vi "多参数据转列表.vi"(7 "参数名":string, 11 "测量数据块":T1) -> (3 "添加的数组":string[][](array[string]))   [LabVIEW 2016, in "斯坦道仪器.lvlib"]
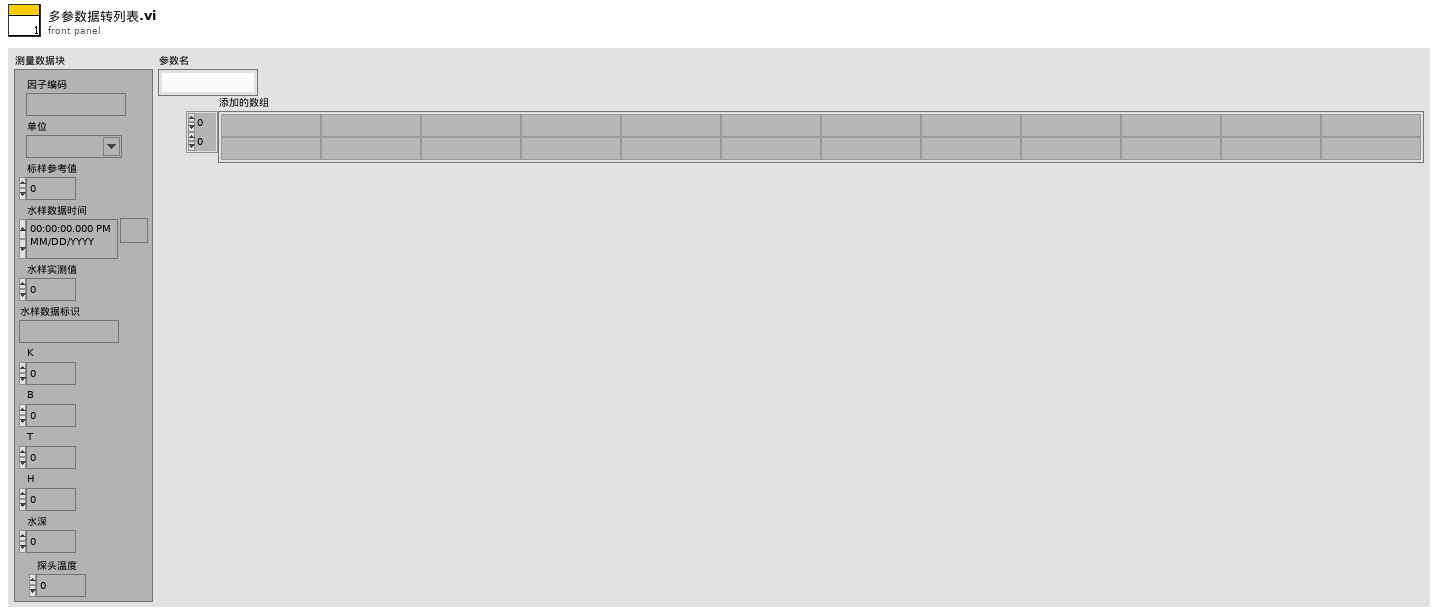
[diagram p1: front panel]
types:
  T1 = cluster{"因子编码":string, "单位":string, "标样参考值":sgl, "水样数据时间":timestamp, "水样实测值":sgl, "水样数据标识":string, "K":sgl, "B":sgl, "T":sgl, "H":sgl, "水深":sgl, "探头温度":sgl}
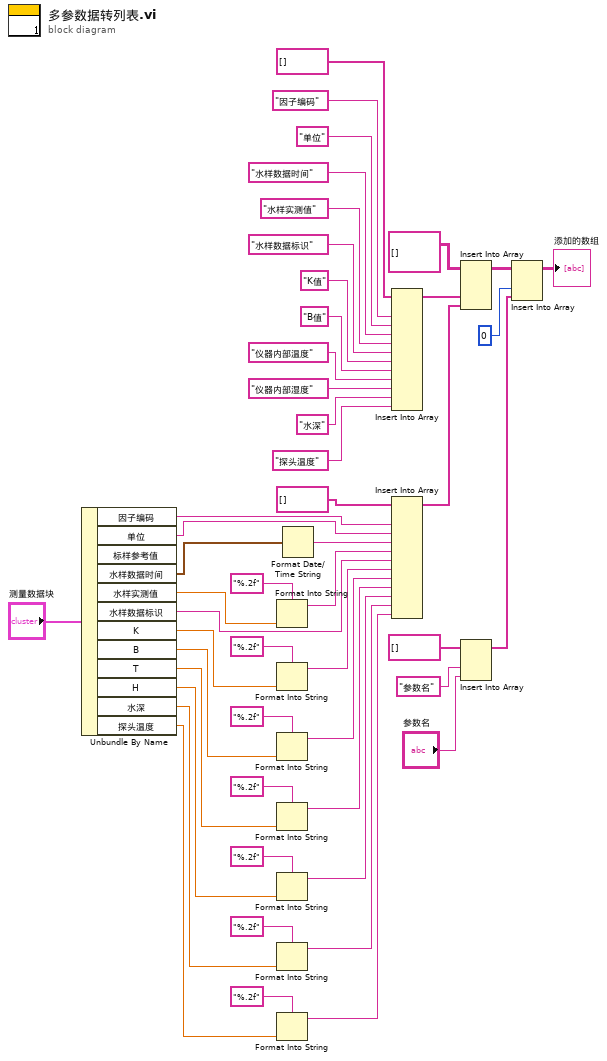
[diagram p0: block diagram]
diagram:
  n1 = Unbundle By Name("测量数据块") -> ("因子编码"=w31:string, "单位"=w30:string, "水样数据时间"=w29:timestamp, "水样实测值"=w28:sgl, "水样数据标识"=w27:string, "K"=w21:sgl, "B"=w20:sgl, "T"=w19:sgl, "H"=w18:sgl, "水深"=w17:sgl, "探头温度"=w2:sgl)  [unwired: 1 out]
  n2 = Format Into String(format string="%.2f" ("格式字符串"), w28) -> (resulting string=w47:string)  [unwired: 2 in, 1 out]
  n3 = Format Into String(format string="%.2f" ("格式字符串"), w21) -> (resulting string=w16:string)  [unwired: 2 in, 1 out]
  n4 = Format Into String(format string="%.2f" ("格式字符串"), w20) -> (resulting string=w15:string)  [unwired: 2 in, 1 out]
  n5 = Format Into String(format string="%.2f" ("格式字符串"), w19) -> (resulting string=w14:string)  [unwired: 2 in, 1 out]
  n6 = Format Into String(format string="%.2f" ("格式字符串"), w18) -> (resulting string=w13:string)  [unwired: 2 in, 1 out]
  n7 = Format Into String(format string="%.2f" ("格式字符串"), w17) -> (resulting string=w12:string)  [unwired: 2 in, 1 out]
  n8 = Format Into String(format string="%.2f" ("格式字符串"), w2) -> (resulting string=w1:string)  [unwired: 2 in, 1 out]
  n9 = Format Date/Time String(seconds (now)=w29) -> (date/time string=w48:string)  [unwired: 2 in]
  n10 = Insert Into Array(array=string[] [], new element #1="因子编码", new element #2="单位", new element #3="水样数据时间", new element #4="水样实测值", new element #5="水样数据标识", new element #6="K值", new element #7="B值", new element #8="仪器内部温度", new element #9="仪器内部湿度", new element #10="水深", new element #11="探头温度") -> (w35:string[])  [unwired: 1 in]
  n11 = Insert Into Array(array=string[] [] ("数组"), new element #1=w31, new element #2=w30, new element #3=w48, new element #4=w47, new element #5=w27, new element #6=w16, new element #7=w15, new element #8=w14, new element #9=w13, new element #10=w12, new element #11=w1) -> (w34:string[])  [unwired: 1 in]
  n12 = Insert Into Array(array=string[][] [], new element #1=w35, new element #2=w34) -> (w11:string[][])  [unwired: 2 in]
  n13 = Insert Into Array(array=string[] [] ("新元素/子数组"), new element #1="参数名" ("新元素/子数组"), new element #2="参数名") -> (w7:string[])  [unwired: 1 in]
  n14 = Insert Into Array(array=w11, index (col)=0 ("禁用的索引 (列)"), new element=w7) -> (→"添加的数组":string[][])  [unwired: 1 in]
